vi "JSON Finalize Configuration.vi"(8 "error in (no error)":errorcluster, 11 "config data":T1) -> (0 "error out":errorcluster, 3 "file json":string)   [LabVIEW 2020, in "DSF Core.lvlib" / "Configuration Session.lvclass"]
uses:
  Configuration Session.lvclass
  Internal DSF Channel Info.ctl
  Internal DSF Channel with ID.ctl
  Internal DSF Transfer Info.ctl
  Internal DSF Transfer with ID.ctl
  Typedefs/DSF Timing Info.ctl
  DSF Core.lvlib
  Internal DSF Group Info.ctl
  Internal DSF Group with ID.ctl
  Typedefs/DSF Settings Info.ctl
  Typedefs/DSF Engine Plugin Thread Configuration.ctl
  Internal DSF Plugin Info.ctl
  Internal DSF Plugin with ID.ctl
  Typedefs/DSF Version Info.ctl
  Internal DSF Settings Info.ctl
  Internal DSF Settings with ID.ctl
  Typedefs/DSF Engine Framework Configuration.ctl
  Internal DSF Configuration.ctl
  Typedefs/DSF Engine Channel Configuration.ctl
  Typedefs/DSF Engine Transfer Configuration.ctl
  Typedefs/DSF Engine Transfer Group Configuration.ctl
  Typedefs/DSF Engine Plugin Configuration.ctl
  Typedefs/DSF Data Type.ctl
  Typedefs/Core Channel Configuration.ctl
  Configuration/Core/Channel/Channel Configuration.lvclass
  Typedefs/Core Transfer Configuration.ctl
  Configuration/Core/Transfer/Transfer Configuration.lvclass
  Typedefs/DSF Direction.ctl
  Typedefs/DSF Timeout Behavior.ctl
  Typedefs/Core Group Configuration.ctl
  Configuration/Core/Group/Group Configuration.lvclass
  Typedefs/Core Thread Configuration.ctl
  Configuration/Core/Thread/Thread Configuration.lvclass
  Typedefs/Core Plugin Configuration.ctl
  Configuration/Core/Plugin/Plugin Configuration.lvclass
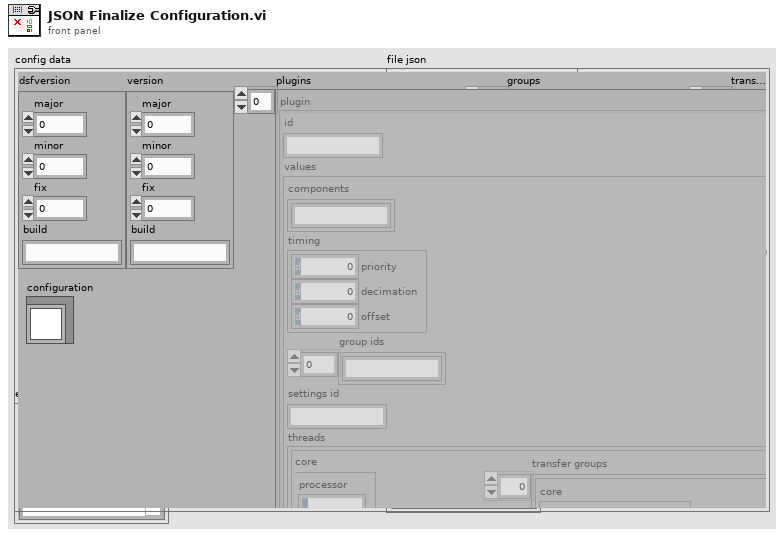
[diagram p1: front panel]
types:
  T1 = typedef "DSF Core.lvlib/Configuration Session.lvclass/Internal DSF Configuration.ctl" = cluster{"dsfversion":T2, "version":T2, "plugins":T3[], "groups":T18[], "transfers":T20[], "channels":T22[], "settings":T24[], "framework configuration":T26, "configuration":refnum<class>}
  T2 = typedef "DSF Core.lvlib/DSF Version Info.ctl" = cluster{"major":u32, "minor":u32, "fix":u32, "build":string}
  T3 = typedef "DSF Core.lvlib/Configuration Session.lvclass/Internal DSF Plugin with ID.ctl" = cluster{"id":string, "values":T4}
  T4 = typedef "DSF Core.lvlib/Configuration Session.lvclass/Internal DSF Plugin Info.ctl" = cluster{"components":string[], "timing":T5, "group ids":string[], "settings id":string, "threads":T6[]}
  T5 = typedef "DSF Core.lvlib/DSF Timing Info.ctl" = cluster{"priority":u64, "decimation":u64, "offset":u64}
  T6 = typedef "DSF Core.lvlib/DSF Engine Plugin Thread Configuration.ctl" = cluster{"core":T7, "component settings":T8[], "transfer groups":T9[]}
  T7 = typedef "DSF Core.lvlib/Thread Configuration.lvclass/Core Thread Configuration.ctl" = cluster{"processor":i32, "priority offset":i16}
  T8 = typedef "DSF Core.lvlib/DSF Settings Info.ctl" = cluster{"component":string, "values":cluster{"key":string, "value":string}[]}
  T9 = typedef "DSF Core.lvlib/DSF Engine Transfer Group Configuration.ctl" = cluster{"core":T10, "component settings":T8[], "transfers":T13[]}
  T10 = typedef "DSF Core.lvlib/Group Configuration.lvclass/Core Group Configuration.ctl" = cluster{"name":string, "direction":T11, "cycle timing":T5, "timeout behavior":T12, "enable conversion":bool}
  T11 = typedef "DSF Core.lvlib/DSF Direction.ctl" = enum8{"Tx", "Rx"}
  T12 = typedef "DSF Core.lvlib/DSF Timeout Behavior.ctl" = enum8{"Increment Late Count", "Throw Error"}
  T13 = typedef "DSF Core.lvlib/DSF Engine Transfer Configuration.ctl" = cluster{"core":T14, "component settings":T8[], "channels":T15[]}
  T14 = typedef "DSF Core.lvlib/Transfer Configuration.lvclass/Core Transfer Configuration.ctl" = cluster{"name":string}
  T15 = typedef "DSF Core.lvlib/DSF Engine Channel Configuration.ctl" = cluster{"core":T16, "component settings":T8[]}
  T16 = typedef "DSF Core.lvlib/Channel Configuration.lvclass/Core Channel Configuration.ctl" = cluster{"name":string, "units":string, "engine data type":T17, "string data type":T17, "string offset":u64}
  T17 = typedef "DSF Core.lvlib/DSF Data Type.ctl" = enum8{"Bool", "SGL", "DBL", "I8", "I16", "I32", "I64", "U8", "U16", "U32", "U64"}
  T18 = typedef "DSF Core.lvlib/Configuration Session.lvclass/Internal DSF Group with ID.ctl" = cluster{"id":string, "values":T19}
  T19 = typedef "DSF Core.lvlib/Configuration Session.lvclass/Internal DSF Group Info.ctl" = cluster{"direction":i32, "timing":T5, "transfer ids":string[], "settings id":string, "thread":i32, "timeout behavior":u8}
  T20 = typedef "DSF Core.lvlib/Configuration Session.lvclass/Internal DSF Transfer with ID.ctl" = cluster{"id":string, "values":T21}
  T21 = typedef "DSF Core.lvlib/Configuration Session.lvclass/Internal DSF Transfer Info.ctl" = cluster{"byte order":i32, "channel ids":string[], "settings id":string}
  T22 = typedef "DSF Core.lvlib/Configuration Session.lvclass/Internal DSF Channel with ID.ctl" = cluster{"id":string, "values":T23}
  T23 = typedef "DSF Core.lvlib/Configuration Session.lvclass/Internal DSF Channel Info.ctl" = cluster{"string buffer offset":u64, "string data type":i32, "engine data type":i32, "settings id":string, "units":string}
  T24 = typedef "DSF Core.lvlib/Configuration Session.lvclass/Internal DSF Settings with ID.ctl" = cluster{"id":string, "values":T25}
  T25 = typedef "DSF Core.lvlib/Configuration Session.lvclass/Internal DSF Settings Info.ctl" = cluster{"key":string, "value":string}[]
  T26 = typedef "DSF Core.lvlib/DSF Engine Framework Configuration.ctl" = cluster{"plugins":T27[]}
  T27 = typedef "DSF Core.lvlib/DSF Engine Plugin Configuration.ctl" = cluster{"core":T28, "component settings":T8[], "threads":T6[]}
  T28 = typedef "DSF Core.lvlib/Plugin Configuration.lvclass/Core Plugin Configuration.ctl" = cluster{"name":string, "components":string[], "cycle timing":T5}
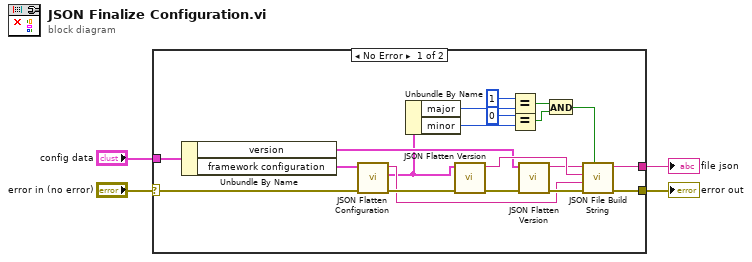
[diagram p0: block diagram]
diagram:
  n1 = case shown="No Error" "error in (no error)" {
    selector: "error in (no error)" -> [w17 w25]
    tunnel: "config data" -> [w24 _]
    tunnel: [w19 w25] -> w3
    tunnel: [w18 _] -> w2
    frame No Error {
      n2 = Unbundle By Name(w24) -> ("version"=w14:T2, "framework configuration"=w23:T26)
      n3 = call "JSON Flatten Configuration.vi"("error in (no error)"=w17, "configuration"=w23) -> ("error out"=w22:errorcluster, "actual file version"=w12:T2, "configuration json"=w16:string)  [unwired: 7 in]
      n4 = Unbundle By Name(w12) -> ("major"=w11:u32, "minor"=w8:u32)
      n5 = call "JSON Flatten Version.vi"("error in (no error)"=w22, "version"=w12) -> ("error out"=w21:errorcluster, "version json"=w15:string)  [unwired: 8 in]
      n6 = Equal?(x=u32 1, y=w11) -> (x = y?=w7:bool)
      n7 = Equal?(x=u32 0, y=w8) -> (x = y?=w6:bool)
      n8 = call "JSON Flatten Version.vi"("error in (no error)"=w21, "version"=w14) -> ("error out"=w20:errorcluster, "version json"=w13:string)  [unwired: 8 in]
      n9 = And(x=w7, y=w6) -> (x .and. y?=w5:bool)
      n10 = call "JSON File Build String.vi"("1.0? (F)"=w5, "error in (no error)"=w20, "dsf configuration substring"=w16, "dsf version substring"=w15, "version substring"=w13) -> ("error out"=w19:errorcluster, "file json string"=w18:string)  [unwired: 5 in]
    }
    frame Error {
    }
  }
  "file json" <- w2
  "error out" <- w3
